vi "SMSLD cRIO Main.vi"() -> ()   [LabVIEW 2014]
doc: "This example runs a background service that initializes and interacts with the Tag Bus Data framework. The service is designed to run continuously so that the framework can be reinitialized with a new configuration without rebooting the target. This can save time when iterating on a configuration.\n\nThe example includes a collection of VIs for sending and receiving messages from the engine service."
uses:
  SubVIs/command commands to rtexe process.ctl
  SubVIs/engine status data.ctl
  <vilib>/NI/Module Execution Interface/Engine Runtime/Execution States.ctl
  <vilib>/NI/Module Execution Interface/Engine Runtime/Fault.ctl
  <vilib>/NI/Tag Bus Module Framework/runtime/error classification.ctl
  SubVIs/queue name.ctl
  <vilib>/NI/AMC/Read Termination Message.vi
  SubVIs/command to string.vi
  SubVIs/string to commands.vi
  <vilib>/NI/AMC/Create Single Message.vi
  <vilib>/NI/AMC/Globals.vi
  SMSLD TBD execution service.lvlib
  <vilib>/NI/AMC/AMC.lvlib
  <vilib>/NI/Module Execution Interface/Engine Runtime/Engine Runtime Interface.lvclass
  <vilib>/NI/Tag Bus Module Framework/runtime/TBM module execution interface.lvclass
panel:
  in  "target alias":string="cRIO"
  in  "Exit":bool
  in  "Reload":bool
  out "final error":errorcluster
  out "system error":errorcluster
  out "engine statuses":T1[](array[typedef])
  out "command error":errorcluster
  out "recent command":T5
  out "engine loaded":string
  out "load error":errorcluster
  out "invalid message":string
  in  "config. file path":path=path "/home/lvuser/natinst/bin/FullSystem.pcfg"
  # "status information"
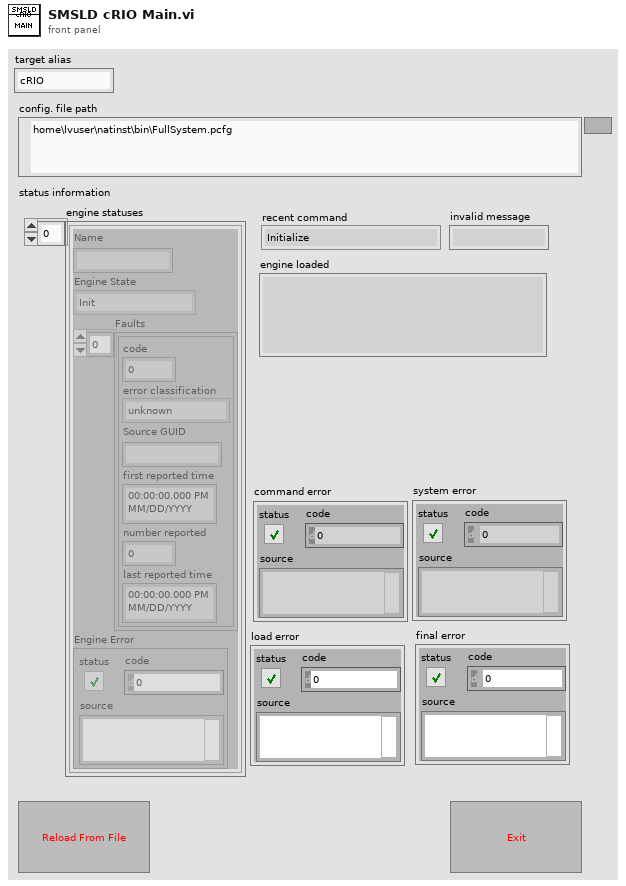
[diagram p1: front panel]
types:
  T1 = typedef "SMSLD TBD execution service.lvlib/engine status data.ctl" = cluster{"Name":string, "Engine State":T2, "Faults":T3[], "Engine Error":errorcluster}
  T2 = typedef "Engine Runtime Interface.lvclass/Execution States.ctl" = enum16{"Init", "Pre-Operational", "Safe-Operational", "Operational", "Stopped"}
  T3 = typedef "Engine Runtime Interface.lvclass/Fault.ctl" = cluster{"code":i32, "error classification":T4, "Source GUID":string, "first reported time":timestamp, "number reported":u32, "last reported time":timestamp}
  T4 = typedef "TBM module execution interface.lvclass/error classification.ctl" = enum16{"unknown", "none", "trivial", "recoverable", "critical"}
  T5 = typedef "SMSLD TBD execution service.lvlib/command commands to rtexe process.ctl" = enum16{"Initialize", "Add Search Paths", "Load from File", "Unload File", "Open All Engines", "Open Single Engine", "Initialize All Engines", "Initialize Single Engine", "Start All", "Start Single", "Pause All", "Pause Single", "Stop All", "Stop Single", "Close All", "Close Single", "Set Safe State All", "Set Safe State Single", "Get Status", "Exit", "Error", "Load Bitfile", "Unload Bitfile", "Clear Faults Single", "Clear Faults All"}
  T6 = typedef "SMSLD TBD execution service.lvlib/queue name.ctl" = enum16{"TOrtmainexec", "FROMrtmainexec"}
  T7 = typedef "AMC.lvlib/Message Queue.ctl" = refnum<queue>
  T8 = typedef "SMSLD TBD execution service.lvlib/common reponses to network process.ctl" = enum16{"System Error", "Load Report", "Action Response", "Engine Status"}
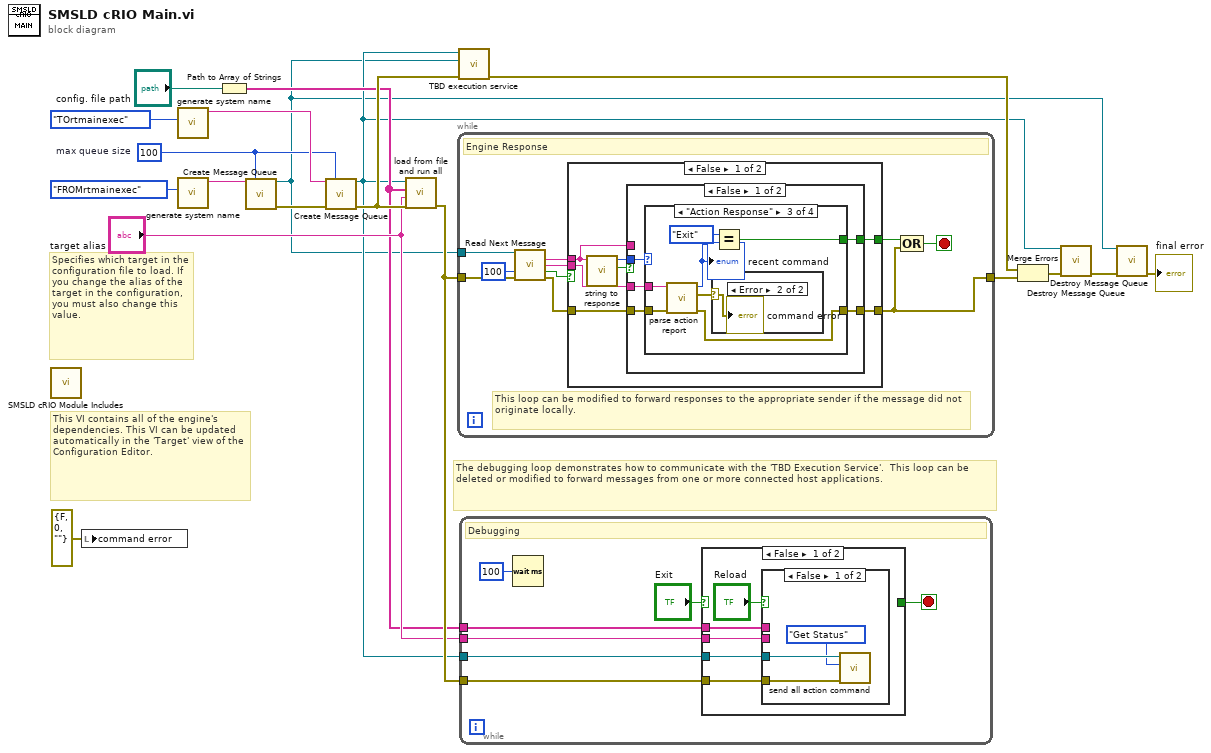
[diagram p0: block diagram]
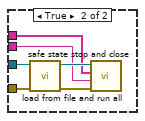
[diagram p2: hidden frame]
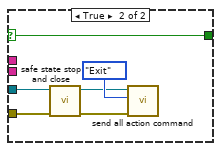
[diagram p3: hidden frame]
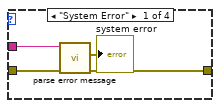
[diagram p4: hidden frame]
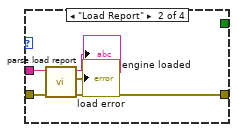
[diagram p5: hidden frame]
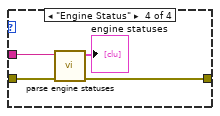
[diagram p7: hidden frame]
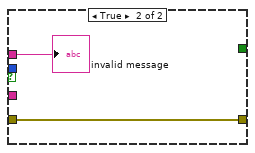
[diagram p8: hidden frame]
diagram:
  w13 = 100  # max queue size
  # "This VI contains all of the engine's dependencies. This VI can be updated automatically in the 'Target' view of the Configuration Editor."
  # "Specifies which target in the configuration file to load. If you change the alias of the target in the configuration, you must also change this value."
  # "The debugging loop demonstrates how to communicate with the 'TBD Execution Service'.  This loop can be deleted or modified to forward messages from one or more connected host applications."
  n1 = call "SMSLD cRIO Module Includes.vi"() -> ()  [unwired: 12 in]
  n2 = local write "command error"(errorcluster {"status"=FALSE, "code"=0, "source"=""} ("command error")) -> ()
  n3 = call "generate system name.vi"("queue type"=queue_name."TOrtmainexec" ("queue")) -> ("queue name"=w17:string)  [unwired: 10 in]
  n4 = call "generate system name.vi"("queue type"=queue_name."FROMrtmainexec" ("queue")) -> ("queue name"=w19:string)  [unwired: 10 in]
  n5 = Path to Array of Strings(0:"config. file path") -> (2:w9:string[])  [unwired: 1 out]
  n6 = call <vilib>:"Create Message Queue.vi"("message queue name"=w19, "max queue size (-1, unlimited)"=w13) -> ("message queue out"=w2:T7, "error out"=w18:errorcluster)  [unwired: 12 in]
  n7 = call <vilib>:"Create Message Queue.vi"("message queue name"=w17, "max queue size (-1, unlimited)"=w13, "error in"=w18) -> ("message queue out"=w3:T7, "error out"=w12:errorcluster)  [unwired: 11 in]
  n8 = call "load from file and run all.vi"("error in"=w12, "target alias"="target alias", "tokenized path"=w9, "message queue in"=w3) -> ("error out"=w11:errorcluster)  [unwired: 6 in, 1 out]
  n9 = while {
    tunnel: w2 -> [w28]
    tunnel: w11 -> [w25]
    tunnel: [w20] -> w8
    stop <- w22 stop-if-true
    # "This loop can be modified to forward responses to the appropriate sender if the message did not originate locally."
    # "Engine Response"
    n10 = call <vilib>:"Read Next Message.vi"("message queue in"=w28, "timeout (1 ms)"=100, "error in"=w25) -> ("message name"=w27:string, "message value"=w21:string, "timed out?"=w24:bool, "error out"=w26:errorcluster)  [unwired: 5 in, 4 out]
    n11 = case shown="False" w24 {
      tunnel: w27 -> [w30 _]
      tunnel: [w35 _] -> w23
      tunnel: w26 -> [w33 w65]
      tunnel: [w32 w65] -> w20
      tunnel: w21 -> [w31 _]
      frame False {
        n12 = call "string to response.vi"("command string"=w30) -> ("invalid"=w36:bool, "responses"=w34:T8)  [unwired: 9 in]
        n13 = case shown="False" w36 {
          tunnel: w31 -> [w40 _]
          tunnel: [w37 _] -> w35
          tunnel: w34 -> [w41 _]
          tunnel: w33 -> [w39 w64]
          tunnel: [w38 w64] -> w32
          tunnel: w30 -> [_ w63]
          frame False {
            n14 = case shown="\"Action Response\"" w41 {
              tunnel: w40 -> [w45 w50 w57 w62]
              tunnel: w39 -> [w44 w49 w56 w61]
              tunnel: [w42 w46 w51 w60] -> w38
              tunnel: [_ _ w53 _] -> w37
              frame "System Error" {
                n15 = call "parse error message.vi"("error in"=w44, "message data"=w45) -> ("error out"=w42:errorcluster, "system error"=→"system error":errorcluster)  [unwired: 8 in]
              }
              frame "Load Report" {
                n16 = call "parse load report.vi"("error in"=w49, "message data"=w50) -> ("error out"=w46:errorcluster, "load error"=→"load error":errorcluster, "engine loaded"=→"engine loaded":string)  [unwired: 7 in]
              }
              frame "Action Response" {
                n17 = call "parse action report.vi"("error in"=w56, "message data"=w57) -> ("error out"=w51:errorcluster, "command error"=w52:errorcluster, "commands"=w55:T5)  [unwired: 7 in]
                "recent command" <- w55
                n18 = case shown="Error" w52 {
                  selector: w52 -> [_ w58]
                  frame No Error {
                  }
                  frame Error {
                    "command error" <- w58
                  }
                }
                n19 = Equal?(x=command_commands_to_rtexe_process."Exit", y=w55) -> (x = y?=w53:bool)
              }
              frame "Engine Status" {
                n20 = call "parse engine statuses.vi"("error in"=w61, "message data"=w62) -> ("error out"=w60:errorcluster, "engine statuses"=→"engine statuses":T1[])  [unwired: 8 in]
              }
            }
          }
          frame True {
            "invalid message" <- w63
          }
        }
      }
      frame True {
      }
    }
    n21 = Compound Arithmetic op=OR(w23, w20) -> (w22:bool)
  }
  n22 = call "TBD execution service.vi"("error in"=w12, "response queue"=w2, "command queue"=w3) -> ("error out"=w7:errorcluster)  [unwired: 8 in]
  n23 = while {
    tunnel: w11 -> [w70]
    tunnel: w3 -> [w71]
    tunnel: w9 -> [w69]
    tunnel: "target alias" -> [w68]
    stop <- w67 stop-if-true
    # "Debugging"
    n24 = Wait (ms)(milliseconds to wait=u32 100) -> ()  [unwired: 1 out]
    n25 = case shown="False" "Exit" {
      selector: "Exit" -> [_ w90]
      tunnel: w71 -> [w76 w92]
      tunnel: w70 -> [w75 w91]
      tunnel: w69 -> [w74 _]
      tunnel: w68 -> [w73 _]
      tunnel: [_ w90] -> w67
      frame False {
        n26 = case shown="False" "Reload" {
          tunnel: w76 -> [w80 w86]
          tunnel: w75 -> [w79 w85]
          tunnel: w74 -> [_ w82]
          tunnel: w73 -> [_ w81]
          frame False {
            n27 = call "send all action command.vi"("error in"=w79, "commands"=command_commands_to_rtexe_process."Get Status", "message queue in"=w80) -> ()  [unwired: 7 in, 2 out]
          }
          frame True {
            n28 = call "safe state stop and close.vi"("error in"=w85, "message queue in"=w86) -> ("error out"=w83:errorcluster, "message queue out"=w84:T7)  [unwired: 8 in]
            n29 = call "load from file and run all.vi"("error in"=w83, "target alias"=w81, "tokenized path"=w82, "message queue in"=w84) -> ()  [unwired: 6 in, 2 out]
          }
        }
      }
      frame True {
        n30 = call "safe state stop and close.vi"("error in"=w91, "message queue in"=w92) -> ("error out"=w87:errorcluster, "message queue out"=w88:T7)  [unwired: 8 in]
        n31 = call "send all action command.vi"("error in"=w87, "commands"=command_commands_to_rtexe_process."Exit", "message queue in"=w88) -> ()  [unwired: 7 in, 2 out]
      }
    }
  }
  n32 = Merge Errors(w7, w8) -> (w4:errorcluster)
  n33 = call <vilib>:"Destroy Message Queue.vi"("message queue in"=w3, "error in"=w4) -> ("error out"=w6:errorcluster)  [unwired: 11 in, 2 out]
  n34 = call <vilib>:"Destroy Message Queue.vi"("message queue in"=w2, "error in"=w6) -> ("error out"=→"final error":errorcluster)  [unwired: 11 in, 2 out]
